vi "Create ZMQ Socket.vi"(8 "error in (no error)":errorcluster, 11 "NewSocket in":refnum<class "NewSocket.lvclass">) -> (0 "error out":errorcluster, 3 "NewSocket out":refnum<class "NewSocket.lvclass">)   [LabVIEW 2018, in "NewSocket.lvclass"]
uses:
  NewSocket.lvclass
  NewSocket.lvclass/NewSocket.ctl
  <vilib>/addons/zeromq/zmq_context.lvclass
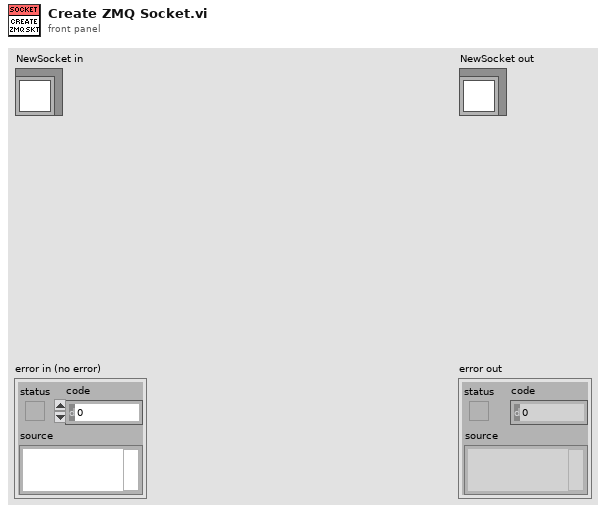
[diagram p1: front panel]
types:
  T1 = typedef "zeromq.lvlib/socket_type.ctl" = enum8{"ZMQ_PAIR", "ZMQ_PUB", "ZMQ_SUB", "ZMQ_REQ", "ZMQ_REP", "ZMQ_DEALER", "ZMQ_ROUTER", "ZMQ_PULL", "ZMQ_PUSH", "ZMQ_XPUB", "ZMQ_XSUB", "ZMQ_STREAM", "ZMQ_SERVER", "ZMQ_CLIENT", "ZMQ_RADIO", "ZMQ_DISH", "ZMQ_GATHER", "ZMQ_SCATTER", "ZMQ_DGRAM"}
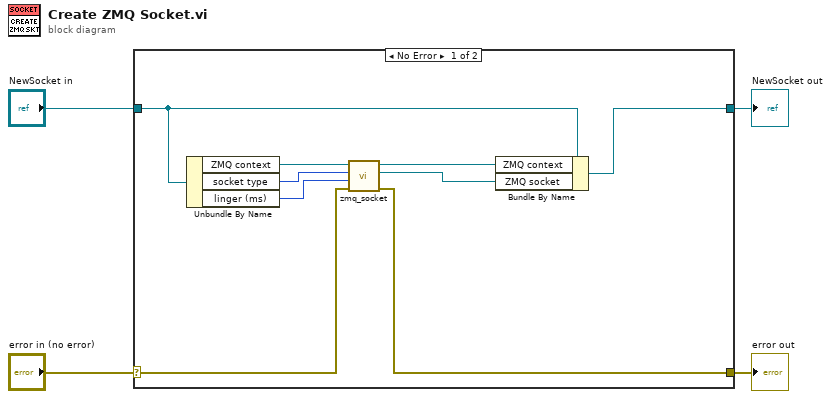
[diagram p0: block diagram]
diagram:
  n1 = case shown="No Error" "error in (no error)" {
    selector: "error in (no error)" -> [w10 w15]
    tunnel: [w9 w15] -> w3
    tunnel: [w7 w14] -> w1
    tunnel: "NewSocket in" -> [w8 w14]
    frame No Error {
      n2 = Unbundle By Name(w8) -> ("ZMQ context"=w13:refnum<class "zmq_context.lvclass">, "socket type"=w12:T1, "linger (ms)"=w11:i32)
      n3 = call <vilib>:"zmq_socket.vi"("error in"=w10, "linger (ms)"=w11, "socket type"=w12, "context in"=w13) -> ("error out"=w9:errorcluster, "socket out"=w5:refnum<class "zmq_socket.lvclass">, "context out"=w6:refnum<class "zmq_context.lvclass">)  [unwired: 1 in]
      n4 = Bundle By Name(cluster=w8, "ZMQ context"=w6, "ZMQ socket"=w5) -> (w7:refnum<class "NewSocket.lvclass">)
    }
    frame Error {
    }
  }
  "error out" <- w3
  "NewSocket out" <- w1
